vi "替换数组成员.vi"() -> ()   [LabVIEW 2010]
panel:
  out "被替换后\n的数组":dbl[][](array[numeric]) format="%.2f"
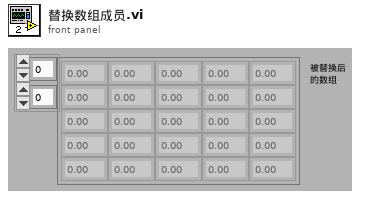
[diagram p1: front panel]
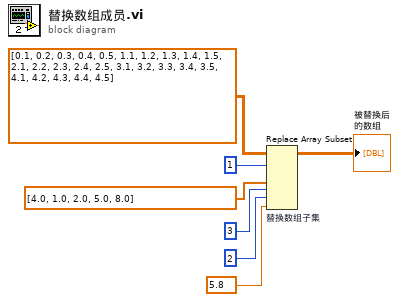
[diagram p0: block diagram]
diagram:
  n1 = Replace Array Subset "替换数组子集"(array=dbl[][] [[0.1, 0.2, 0.3, 0.4, 0.5], [1.1, 1.2, 1.3, 1.4, 1.5], [2.1, 2.2, 2.3, 2.4, 2.5], [3.1, 3.2, 3.3, 3.4, 3.5], [4.1, 4.2, 4.3, 4.4, 4.5]], new element #1=dbl[] [4.0, 1.0, 2.0, 5.0, 8.0], index (row) #1=1 ("index (row)"), new element #2=5.8 ("new element/subarray"), index (row) #2=3 ("index (row)"), index (col) #2=2 ("disabled index (col)")) -> (→"被替换后\n的数组":dbl[][])  [unwired: 1 in]
